vi "file header.vi"(8 "error in (no error)":errorcluster, 11 "Log File in":refnum<class "CM_Log File.lvclass">) -> (0 "error out":errorcluster, 3 "Log File out":refnum<class "CM_Log File.lvclass">)   [LabVIEW 2018, in "CM_Log File.lvclass"]
uses:
  CM_Log File.lvclass
  CM_Log File.lvclass/CM_Log File.ctl
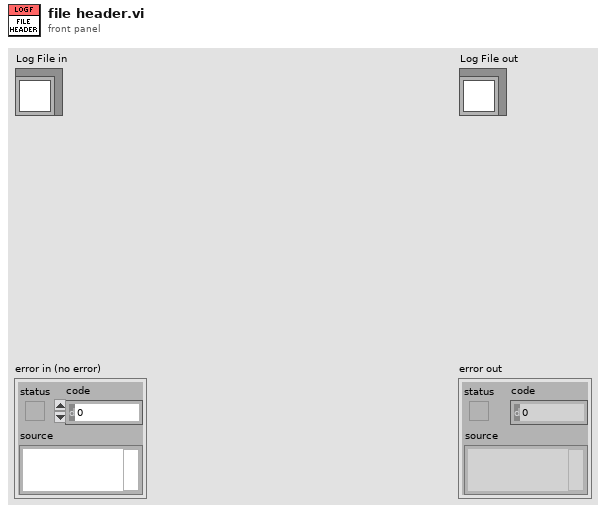
[diagram p1: front panel]
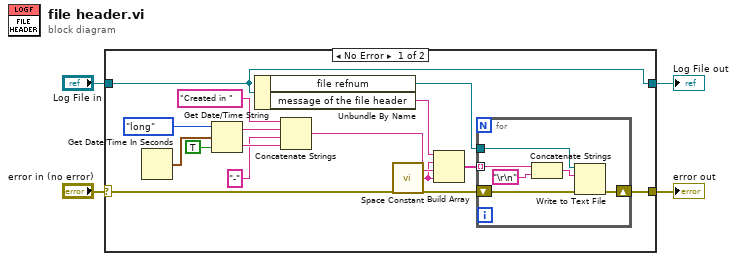
[diagram p0: block diagram]
diagram:
  n1 = case shown="No Error" "error in (no error)" {
    selector: "error in (no error)" -> [w17 w27]
    tunnel: [w16 w27] -> w3
    tunnel: [w19 w26] -> w1
    tunnel: "Log File in" -> [w19 w26]
    frame No Error {
      n2 = Get Date/Time In Seconds() -> (seconds since 1Jan1904=w14:timestamp)
      n3 = Get Date/Time String(date format (0)=enum16{"short", "long", "abbreviated"}."long", seconds (now)=w14, want seconds? (F)=TRUE) -> (date string=w13:string, time string=w12:string)
      n4 = Unbundle By Name(w19) -> ("file refnum"=w18:refnum<file>, "message of the file header"=w7:string)
      n5 = Concatenate Strings("Created in ", w13, "-" ("string"), w12) -> (w6:string)
      n6 = call <vilib>:"Space Constant.vi"() -> ("String"=w5:string)
      n7 = Build Array(w7, w5, w6, w5) -> (w15:string[])
      n8 = for {
        tunnel: w18 -> [w25]
        shift-right: [w23] -> w16
        shift-left: w17 -> [w24]
        tunnel: w15 -> [w22] mode=indexing
        n9 = Concatenate Strings(w22, "\r\n") -> (w20:string)
        n10 = Write to Text File(file (use dialog)=w25, text=w20, error in=w24) -> (error out=w23:errorcluster)  [unwired: 1 in, 2 out]
      }
    }
    frame Error {
    }
  }
  "error out" <- w3
  "Log File out" <- w1
